vi "LoadGeneralConfigData.vi"(8 "error in (no error)":errorcluster, 11 "configuration file path":path) -> (0 "error out":errorcluster, 1 "Config Cluster":T1, 3 "Refnum out":T2)   [LabVIEW 2014]
uses:
  <vilib>/Utility/config.llb/Config Data RefNum.ctl
  <vilib>/Utility/config.llb/Read Key (Double).vi
  <vilib>/Utility/config.llb/Read Key (I32).vi
  Variables/Global.vi
  <vilib>/Utility/config.llb/NI_LVConfig.lvlib
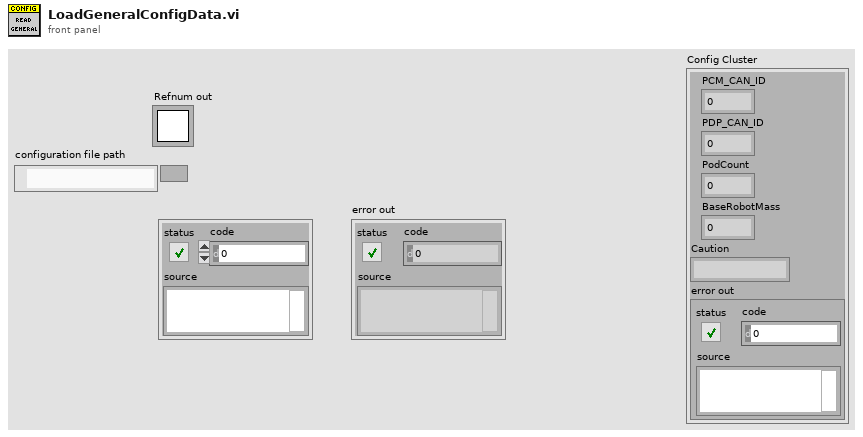
[diagram p1: front panel]
types:
  T1 = cluster{"PCM_CAN_ID":dbl, "PDP_CAN_ID":dbl, "PodCount":dbl, "BaseRobotMass":dbl, "Caution":string, "error out":errorcluster}
  T2 = typedef "NI_LVConfig.lvlib/Config Data RefNum.ctl" = refnum<k1>
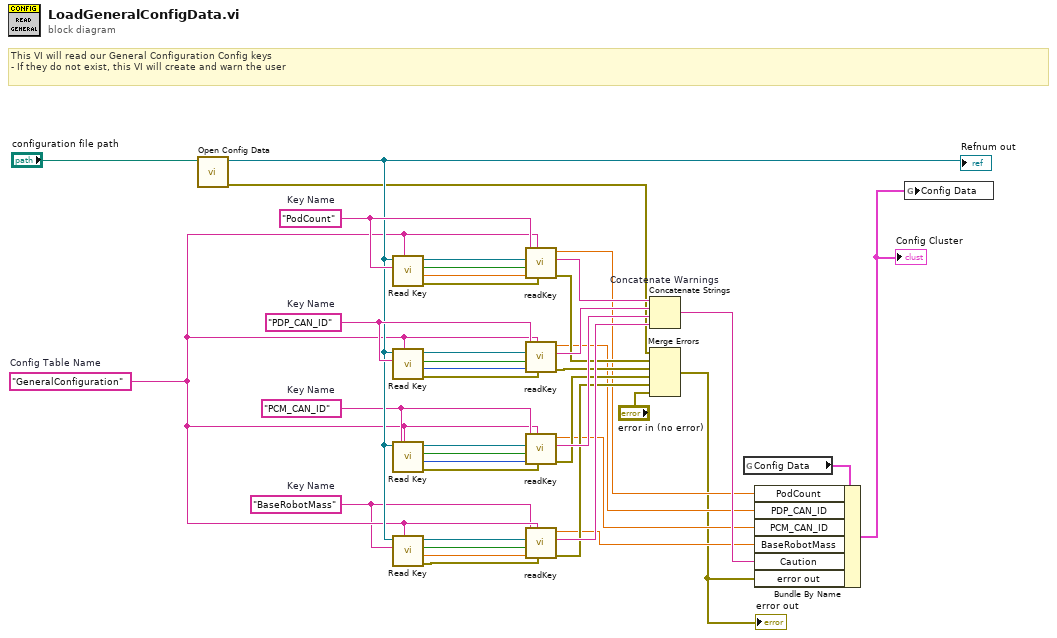
[diagram p0: block diagram]
diagram:
  w23 = "BaseRobotMass"  # Key Name
  w24 = "GeneralConfiguration"  # Config Table Name
  w25 = "PCM_CAN_ID"  # Key Name
  w31 = "PDP_CAN_ID"  # Key Name
  w32 = "PodCount"  # Key Name
  # "This VI will read our General Configuration Config keys\n- If they do not exist, this VI will create and warn the user"
  n1 = call <vilib>:"Open Config Data.vi"("configuration file path"="configuration file path") -> ("error out"=w1:errorcluster, "refnum"=w26:T2)  [unwired: 8 in, 1 out]
  "Refnum out" <- w26
  n2 = call-poly <vilib>:"Read Key.vi"("section"=w24, "key"=w32, "refnum"=w26) -> ("error out"=w35:errorcluster, "value"=w36:dbl, "found?"=w34:bool, "refnum out"=w33:T2)  [unwired: 5 in]
  n3 = call-poly <vilib>:"Read Key.vi"("section"=w24, "key"=w31, "refnum"=w26) -> ("error out"=w27:errorcluster, "value"=w28:i32, "found?"=w29:bool, "refnum out"=w30:T2)  [unwired: 5 in]
  n4 = call-poly <vilib>:"Read Key.vi"("section"=w24, "key"=w25, "refnum"=w26) -> ("error out"=w15:errorcluster, "value"=w19:i32, "found?"=w20:bool, "refnum out"=w21:T2)  [unwired: 5 in]
  n5 = call-poly <vilib>:"Read Key.vi"("section"=w24, "key"=w23, "refnum"=w26) -> ("error out"=w16:errorcluster, "value"=w17:dbl, "found?"=w18:bool, "refnum out"=w22:T2)  [unwired: 5 in]
  n6 = call "readKey.vi"("Error in"=w35, "Table Name"=w24, "Value"=w36, "Found?"=w34, "Refnum in"=w33, "Key Name"=w32) -> ("error out"=w11:errorcluster, "Warning"=w39:string, "value"=w4:dbl)  [unwired: 3 in]
  n7 = call "readKey.vi"("Error in"=w27, "Table Name"=w24, "Value"=w28, "Found?"=w29, "Refnum in"=w30, "Key Name"=w31) -> ("error out"=w10:errorcluster, "Warning"=w14:string, "value"=w7:dbl)  [unwired: 3 in]
  n8 = call "readKey.vi"("Error in"=w15, "Table Name"=w24, "Value"=w19, "Found?"=w20, "Refnum in"=w21, "Key Name"=w25) -> ("error out"=w9:errorcluster, "Warning"=w13:string, "value"=w6:dbl)  [unwired: 3 in]
  n9 = call "readKey.vi"("Error in"=w16, "Table Name"=w24, "Value"=w17, "Found?"=w18, "Refnum in"=w22, "Key Name"=w23) -> ("error out"=w8:errorcluster, "Warning"=w12:string, "value"=w5:dbl)  [unwired: 3 in]
  n10 = Concatenate Strings "Concatenate Warnings"(w39, w14, w13, w12) -> (w38:string)
  n11 = Merge Errors "Merge Errors"(w1, w11, w10, w9, w8, "error in (no error)") -> (w3:errorcluster)
  "error out" <- w3
  n12 = global read "Global.vi" "Config Data"() -> (w41:T1)
  n13 = Bundle By Name(cluster=w41, "PodCount"=w4, "PDP_CAN_ID"=w7, "PCM_CAN_ID"=w6, "BaseRobotMass"=w5, "Caution"=w38, "error out"=w3) -> (w40:T1)
  "Config Cluster" <- w40
  n14 = global write "Global.vi" "Config Data"(w40) -> ()
